vi "Get Index.vi"(8 "error in (no error)":errorcluster, 11 "ODentry in":refnum<class "ODentry.lvclass">) -> (0 "error out":errorcluster, 2 "Index":u16, 3 "ODentry out":refnum<class "ODentry.lvclass">)   [LabVIEW 2024, in "EDS.lvlib" / "ODentry.lvclass"]
uses:
  ODentry.lvclass
  ODentry.lvclass/ODentry.ctl
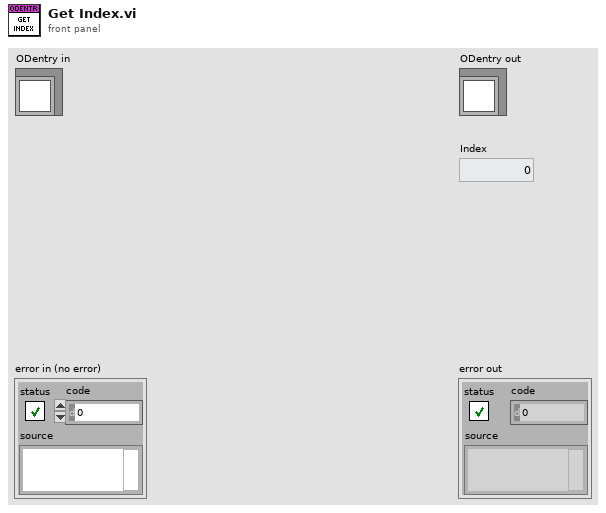
[diagram p1: front panel]
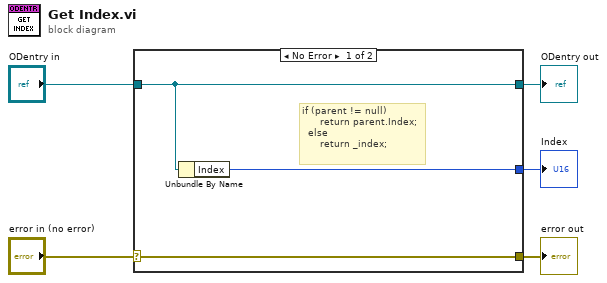
[diagram p0: block diagram]
diagram:
  n1 = case shown="No Error" "error in (no error)" {
    selector: "error in (no error)" -> [w8 w9]
    tunnel: [w8 w9] -> w4
    tunnel: [w7 w10] -> w2
    tunnel: "ODentry in" -> [w7 w10]
    tunnel: [w6 _] -> w1
    frame No Error {
      # "if (parent != null)\n      return parent.Index;\n  else\n      return _index;"
      n2 = Unbundle By Name(w7) -> ("Index"=w6:u16)
    }
    frame Error {
    }
  }
  "error out" <- w4
  "ODentry out" <- w2
  "Index" <- w1
